vi "TLS Handshake.vi"(8 "error in (no error)":errorcluster, 11 "Websocket Client in":refnum<class "Websocket Client.lvclass">) -> (0 "error out":errorcluster, 3 "Websocket Client out":refnum<class "Websocket Client.lvclass">)   [LabVIEW 2020, in "Stream-Websocket.lvlib" / "Websocket Client.lvclass"]
uses:
  Websocket Client.lvclass
  C:/dev/lv20CE/relink/lv-stream/stream/Endpoint/Endpoint.lvclass
  Websocket Client.lvclass/Websocket Client.ctl
  lv-stream/stream/Endpoint/Endpoint.lvclass
  lv-stream/stream/URI/URI.lvclass
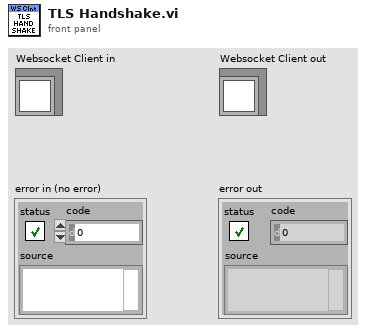
[diagram p1: front panel]
types:
  T1 = typedef "Stream-Websocket.lvlib/Websocket Client.lvclass/Ref Data.ctl" = cluster{"TCP Connection":refnum<k5>, "WS Stream":refnum<class "WebsocketStream.lvclass">, "Connection Loop":refnum<vi>, "Timeout ms":i32, "Server Connection":bool}
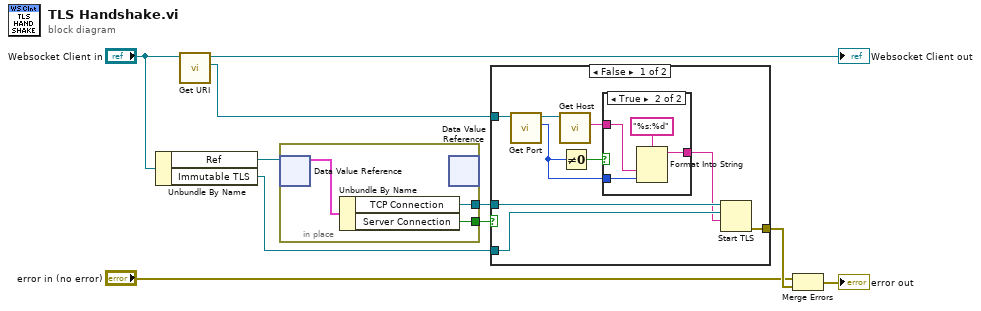
[diagram p0: block diagram]
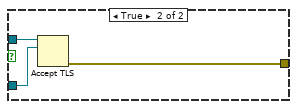
[diagram p3: hidden frame]
diagram:
  n1 = Unbundle By Name("Websocket Client in") -> ("Ref"=w9:refnum<data-value>, "Immutable TLS"=w10:refnum<k36>)
  n2 = call "Get URI.vi"("Endpoint in"="Websocket Client in") -> ("URI"=w7:refnum<class "URI.lvclass">, "Endpoint out"=→"Websocket Client out":refnum<class "Websocket Client.lvclass">)  [unwired: 8 in, 1 out]
  n3 = in-place {
    in-place-border: [w12] -> w2
    in-place-border: [w11] -> w1
    n4 = in-place-dvr #1(w9) -> (w13:T1)  [unwired: 1 out]
    n5 = Unbundle By Name(w13) -> ("TCP Connection"=w12:refnum<k5>, "Server Connection"=w11:bool)
    n6 = in-place-dvr #1() -> ()  [unwired: 1 in, 2 out]
  }
  n7 = case shown="False" w1 {
    tunnel: w2 -> [w22 w30]
    tunnel: w10 -> [w21 w29]
    tunnel: [w20 w28] -> w5
    tunnel: w7 -> [w19 _]
    frame False {
      n8 = call "Get Port.vi"("URI in"=w19) -> ("Port"=w15:u16, "URI out"=w18:refnum<class "URI.lvclass">)  [unwired: 8 in, 1 out]
      n9 = call "Get Host.vi"("URI in"=w18) -> ("Host"=w17:string)  [unwired: 8 in, 2 out]
      n10 = Not Equal To 0?(x=w15) -> (x != 0?=w14:bool)
      n11 = case shown="True" w14 {
        tunnel: w17 -> [w23 w26]
        tunnel: [w23 w25] -> w16
        tunnel: w15 -> [_ w24]
        frame False {
        }
        frame True {
          n12 = Format Into String(format string="%s:%d", w26, w24) -> (resulting string=w25:string)  [unwired: 2 in, 1 out]
        }
      }
      n13 = Start TLS(9:w16, 10:w21, 11:w22) -> (0:w20:errorcluster)  [unwired: 3 in, 2 out]
    }
    frame True {
      n14 = Accept TLS(10:w29, 11:w30) -> (0:w28:errorcluster)  [unwired: 2 in, 2 out]
    }
  }
  n15 = Merge Errors("error in (no error)", w5) -> (→"error out":errorcluster)
